vi "ImagerForFlowbit.vi"() -> ()   [LabVIEW 2011]
uses:
  <vilib>/Platform/TimedLoop/XDataNode/timing_clust.ctl
  <vilib>/Platform/TimedLoop/XDataNode/nitl_modes.ctl
  <vilib>/Platform/TimedLoop/XDataNode/wakeup.ctl
  <vilib>/Instr/_visa.llb/VISA Configure Serial Port (Instr).vi
  <vilib>/Platform/TimedLoop/XDataNode/XDataNode.xnode
  <vilib>/Platform/TimedLoop/XDataNode/XDNodeRunTimeDep.lvlib
  <vilib>/vision/NI_Vision_Development_Module.lvlib
panel:
  in  "热图":bool
  out "FramesPerStim":i32
  out "停止 4":bool
  in  "停止 3":bool
  in  "recording_temp":bool
  in  "datatype":enum16{"U8", "I16", "U32", "SGL"}(ring)=enum."SGL"
  out "Y Resolution":i32
  out "X Resolution":i32
  in  "frame_count":i32
  out "队列中元素数量":i32(slide) scale=0.0..100.0
  out "当前blk句柄":refnum<file>
  out "Recording":bool
  in  "bin_num":i32=25
  out "错误输出":errorcluster
  in  "BlkFolderPath":path=path "D:/Expt/test"
  out "循环持续时间":i64
  out "Image":T1(plugin-control)
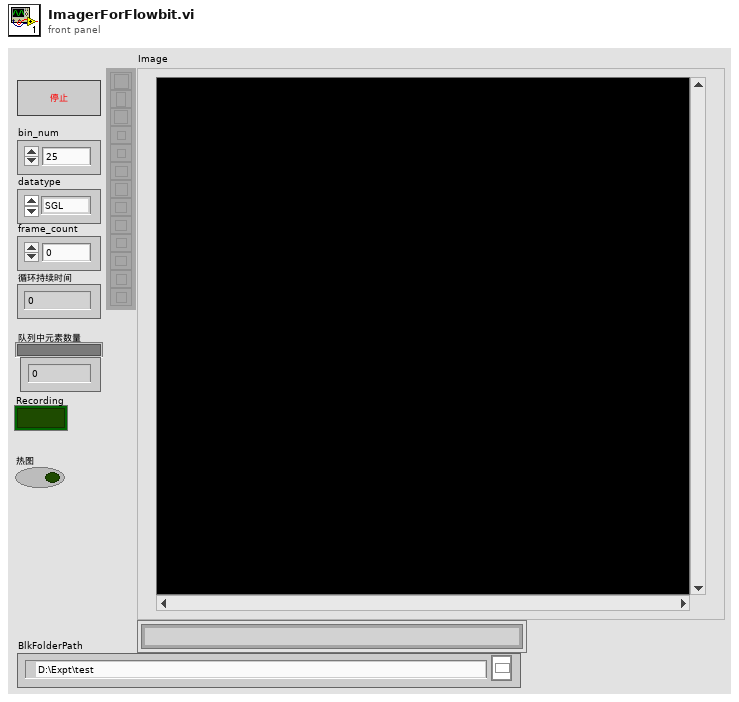
[diagram p1: front panel]
types:
  T1 = typedef "IMAQ Image.ctl" = refnum<image>
  T2 = typedef "Image Type" = u32
  T3 = enum16{"Disable External Trigger", "Enable External Trigger"}
  T4 = enum32{"Auto Detect", "RoadRunner", "Raven", "R64"}
  T5 = enum16{"open", "replace", "create", "open or create", "replace or create", "replace or create with confirmation"}
  T6 = typedef "XDNodeRunTimeDep.lvlib/timing_clust.ctl" = cluster{"Expected End [f-1]":u64, "Actual End [f-1]":u64, "Finished Late? [f-1]":bool, "Expected End [i-1]":u64, "Actual End [i-1]":u64, "Finished Late? [i-1]":bool, "Expected Start [i]":u64, "Actual Start [i]":u64, "Expected Start [f]":u64, "Actual Start [f]":u64, "Source Name":string, "Structure Name":string, "Period":i64, "Deadline":i64, "Offset":i64, "Start":i64, "Priority":i32, "Timeout":i32, "Mode":T7, "Wakeup Reason":T8, "Error":errorcluster, "Source Type":string, "Secondary Source Type":string, "Global End Time":u64, "Global Start Time":u64, "Frame Duration":u64, "Iteration Duration":u64, "Assigned CPU":i32, "I/O Scan Engine Mode":u32}
  T7 = typedef "XDNodeRunTimeDep.lvlib/nitl_modes.ctl" = enum32{"No Change", "Process missed periods, maintain original phase", "Discard missed periods, maintain original phase", "Process missed periods, ignore original phase", "Discard missed periods, ignore original phase"}
  T8 = typedef "XDNodeRunTimeDep.lvlib/wakeup.ctl" = enum32{"Normal", "Aborted", "Asynchronous wakeup", "Timing source error", "Timed loop error", "Timeout"}
  T9 = enum16{"big-endian, network order", "native, host order", "little-endian"}
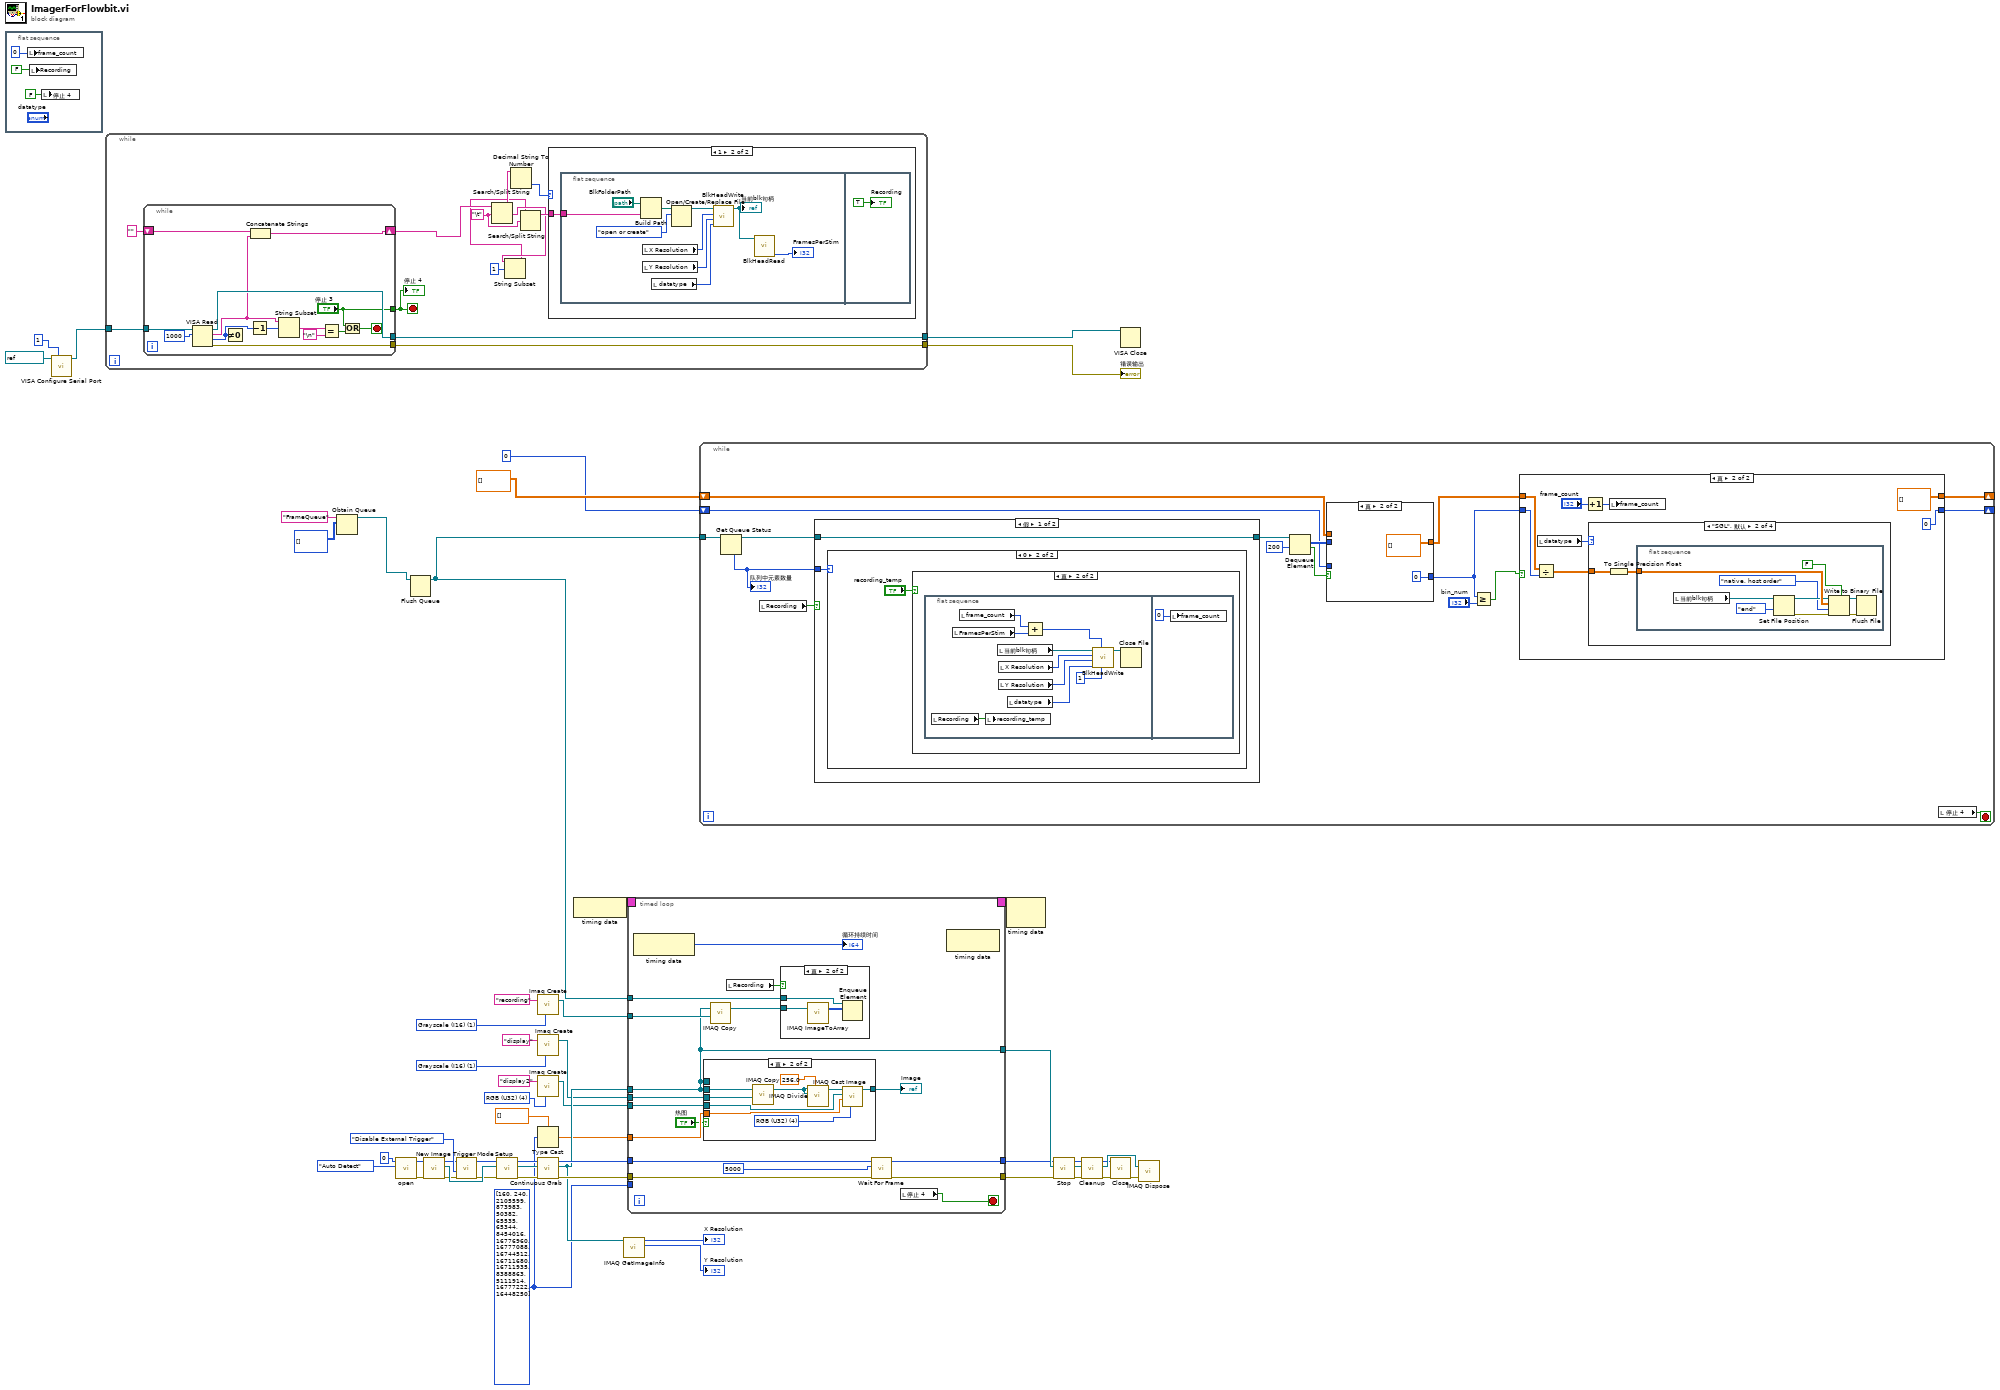
[diagram p0: block diagram]
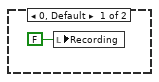
[diagram p2: hidden frame]
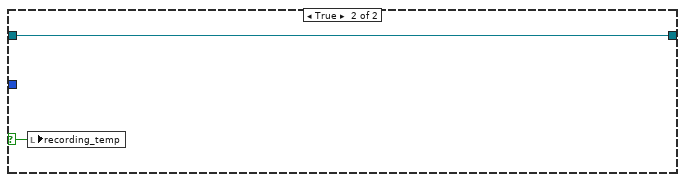
[diagram p7: hidden frame]
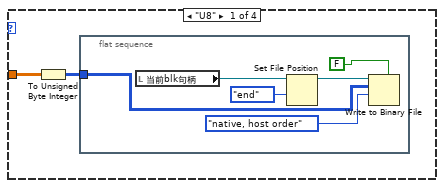
[diagram p9: hidden frame]
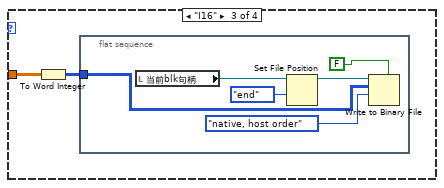
[diagram p10: hidden frame]
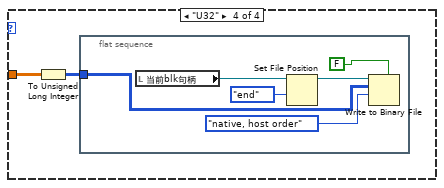
[diagram p11: hidden frame]
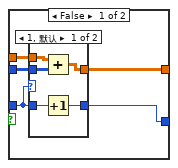
[diagram p12: hidden frame]
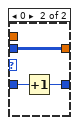
[diagram p13: hidden frame]
diagram:
  w5 = T2 4 items=["Grayscale (U8)", "Grayscale (I16)", "Grayscale (SGL)", "Complex (CSG)", "RGB (U32)", "HSL (U32)", "RGB (U64)", "Grayscale (U16)"] ("Image Type")
  w3 = u32[] [160, 240, 2105599, 873983, 50382, 65535, 65344, 8454016, 16776960, 16777088, 16744512, 16711680, 16711935, 8388863, 5111914, 16777222, 16448250] ("数组")
  w9 = T2 1 items=["Grayscale (U8)", "Grayscale (I16)", "Grayscale (SGL)", "Complex (CSG)", "RGB (U32)", "HSL (U32)", "RGB (U64)", "Grayscale (U16)"] ("Image Type")
  w24 = T2 1 items=["Grayscale (U8)", "Grayscale (I16)", "Grayscale (SGL)", "Complex (CSG)", "RGB (U32)", "HSL (U32)", "RGB (U64)", "Grayscale (U16)"] ("Image Type")
  n1 = flat-sequence {
    frame #0 {
      n2 = local write "frame_count"(0 ("frame_count")) -> ()
      n3 = local write "Recording"(FALSE ("Recording")) -> ()
      n4 = local write "停止 4"(FALSE ("停止 3")) -> ()
    }
  }
  n5 = call-poly "VISA Configure Serial Port"("VISA resource name"=refnum<visa-resource-name> "COM3", "timeout (10sec)"=u32 1) -> ("VISA resource name out"=w22:refnum<visa-resource-name>)  [unwired: 12 in, 1 out]
  n6 = while {
    tunnel: w22 -> [w68]
    tunnel: [w67] -> w20
    tunnel: [w66] -> w19
    stop <- w65 stop-if-true
    w62 = "\t"
    n7 = while {
      tunnel: w68 -> [w95]
      tunnel: [w94] -> w67
      tunnel: [w93] -> w66
      shift-right: [w86] -> w60
      shift-left: "" ("read buffer") -> [w92]
      tunnel: ["停止 3"] -> w65
      stop <- w84 stop-if-true
      n8 = VISA Read(VISA resource name=w95, byte count=u32 1000 ("字节总数")) -> (VISA resource name out=w93:refnum<visa-resource-name>, read buffer=w91:string, return count=w90:u32, error out=w94:errorcluster)  [unwired: 1 in]
      n9 = Not Equal To 0?(x=w90) -> ()  [unwired: 1 out]
      n10 = Decrement(x=w90) -> (x-1=w89:u32)
      n11 = Concatenate Strings(w92, w91) -> (w86:string)
      n12 = String Subset(string=w91, offset (0)=w89) -> (substring=w88:string)  [unwired: 1 in]
      n13 = Equal?(x=w88, y="\n") -> (x = y?=w85:bool)
      n14 = Or(x="停止 3", y=w85) -> (x .or. y?=w84:bool)
    }
    "停止 4" <- w65
    n15 = Search/Split String(string=w60, search string/char (-)=w62) -> (substring before match=w63:string, match + rest of string=w59:string)  [unwired: 1 in, 1 out]
    n16 = String Subset(string=w59, offset (0)=1 ("偏移量(0)")) -> (substring=w57:string)  [unwired: 1 in]
    n17 = Decimal String To Number(string=w63) -> (number=w64:i32)  [unwired: 2 in, 1 out]
    n18 = Search/Split String(string=w57, search string/char (-)=w62) -> (substring before match=w61:string)  [unwired: 1 in, 2 out]
    n19 = case shown="1" w64 {
      tunnel: w61 -> [_ w71]
      frame 0, Default {
        n20 = local write "Recording"(FALSE ("Recording")) -> ()
      }
      frame 1 {
        n21 = flat-sequence {
          tunnel: w71 -> [w75]
          frame #0 {
            n22 = Build Path(base path="BlkFolderPath", name or relative path=w75) -> (appended path=w79:path)
            n23 = local read "X Resolution"() -> (w78:i32)
            n24 = local read "Y Resolution"() -> (w77:i32)
            n25 = local read "datatype"() -> (w76:enum16{"U8", "I16", "U32", "SGL"})
            n26 = Open/Create/Replace File(file path (use dialog)=w79, operation (0:open)=T5."open or create" ("操作(0:open)")) -> (refnum out=w72:refnum<file>)  [unwired: 4 in, 2 out]
            n27 = call "BlkHeadWrite.vi"("datatype"=w76, "FrameHeight"=w77, "FrameWidth"=w78, "BlkFile"=w72) -> ("引用句柄输出"=w74:refnum<file>)  [unwired: 7 in]
            "当前blk句柄" <- w74
            n28 = call "BlkHeadRead.vi"("引用句柄"=w74) -> ("FramesPerStim"=→"FramesPerStim":i32)  [unwired: 5 in, 5 out]
          }
          frame #1 {
            "Recording" <- TRUE ("Recording")
          }
        }
      }
    }
  }
  "错误输出" <- w20
  n29 = Obtain Queue(name (unnamed)="FrameQueue" ("名称（未命名）"), element data type=i16[][] []) -> (queue out=w11:refnum<queue>)  [unwired: 3 in, 2 out]
  n30 = call <vilib>:"open.vi"("Board Type"=T4."Auto Detect", "Board Number"=u32 0) -> ("error out"=w42:errorcluster, "RefBrdOut"=w37:u32)  [unwired: 2 in, 5 out]
  n31 = Flush Queue(queue=w11) -> (queue out=w10:refnum<queue>)  [unwired: 1 in, 2 out]
  n32 = call <vilib>:"New Image.vi"("RefBrdIn"=w37, "error in"=w42) -> ("RefBrdOut"=w36:u32, "Image"=w51:T1, "error out"=w43:errorcluster)  [unwired: 6 in]
  n33 = call <vilib>:"Trigger Mode.vi"("RefBrdIn"=w36, "Trigger Mode"=T3."Disable External Trigger", "error in (no error)"=w43) -> ("RefBrdOut"=w35:u32, "error out"=w44:errorcluster)  [unwired: 6 in]
  n34 = call <vilib>:"Setup.vi"("error in"=w44, "Image In"=w51, "RefBrdIn"=w35) -> ("error out"=w39:errorcluster, "Image"=w40:T1, "RefBrdOut"=w34:u32)  [unwired: 6 in]
  n35 = call "Imaq Create"("Image Name"="recording", "Image Type"=w24) -> ("New Image"=w26:T1)  [unwired: 3 in, 1 out]
  n36 = call "Imaq Create"("Image Name"="display", "Image Type"=w9) -> ("New Image"=w7:T1)  [unwired: 3 in, 1 out]
  n37 = call "Imaq Create"("Image Name"="display2", "Image Type"=w5) -> ("New Image"=w4:T1)  [unwired: 3 in, 1 out]
  n38 = Type Cast(type=sgl[] [] ("单精度浮点"), x=w3) -> (*(type *) &x=w1:sgl[])
  n39 = call <vilib>:"Continuous Grab.vi"("error in (no error)"=w39, "Image In"=w40, "RefBrdIn"=w34) -> ("error out"=w38:errorcluster, "Image"=w14:T1, "RefBrdOut"=w33:u32)  [unwired: 6 in]
  n40 = node-c288() -> (w28:T6)
  n41 = call "IMAQ GetImageInfo"("Image"=w14) -> ("Y Resolution"=→"Y Resolution":i32, "X Resolution"=→"X Resolution":i32)  [unwired: 3 in, 6 out]
  n42 = timed-loop {
    tunnel: [w99] -> w50
    tunnel: [w113] -> w45
    tunnel: w14 -> [w99]
    tunnel: w38 -> [w112]
    tunnel: w33 -> [w111]
    tunnel: [w110] -> w32
    timing: w28 -> [_]
    timing-out: [_] -> w27
    tunnel: w26 -> [w104]
    tunnel: w10 -> [w108]
    tunnel: w7 -> [w102]
    tunnel: w3 -> [_]
    tunnel: w4 -> [w101]
    tunnel: w1 -> [w100]
    stop <- w105 stop-if-true
    n43 = node-c288() -> (→"循环持续时间":i64)  [unwired: 1 in]
    n44 = case shown="真" "热图" {
      tunnel: w102 -> [_ w122]
      tunnel: w99 -> [_ w120]
      tunnel: [w114 w119] -> w98
      tunnel: w101 -> [_ w117]
      tunnel: w100 -> [_ w116]
      tunnel: w99 -> [w114 _]
      frame False {
      }
      frame True {
        w118 = T2 4 items=["Grayscale (U8)", "Grayscale (I16)", "Grayscale (SGL)", "Complex (CSG)", "RGB (U32)", "HSL (U32)", "RGB (U64)", "Grayscale (U16)"] ("Image Type")
        n45 = call "IMAQ Copy"("Image Dst"=w122, "Image Src"=w120) -> ("Image Dst Out"=w121:T1)  [unwired: 4 in, 1 out]
        n46 = call "IMAQ Divide"("Image Src A"=w121, "Constant"=sgl 256.0, "Image Dst"=w121) -> ("Image Dst Out"=w115:T1)  [unwired: 4 in, 1 out]
        n47 = call "IMAQ Cast Image"("Image Type"=w118, "Lookup Table"=w116, "Image Dst"=w117, "Image Src"=w115) -> ("Image Dst Out"=w119:T1)  [unwired: 6 in, 1 out]
      }
    }
    "Image" <- w98
    n48 = call "IMAQ Copy"("Image Dst"=w104, "Image Src"=w99) -> ("Image Dst Out"=w103:T1)  [unwired: 4 in, 1 out]
    n49 = local read "Recording"() -> (w106:bool)
    n50 = case shown="真" w106 {
      tunnel: w108 -> [_ w126]
      tunnel: w103 -> [_ w124]
      frame False {
      }
      frame True {
        n51 = call "IMAQ ImageToArray"("Image"=w124) -> ("Image Pixels (I16)"=w125:i16[][])  [unwired: 3 in, 4 out]
        n52 = Enqueue Element(queue=w126, element=w125) -> ()  [unwired: 2 in, 3 out]
      }
    }
    n53 = call <vilib>:"Wait For Frame.vi"("error in (no error)"=w112, "Timeout (mS)"=u32 5000, "RefBrdIn"=w111) -> ("error out"=w113:errorcluster, "RefBrdOut"=w110:u32)  [unwired: 7 in]
    n54 = local read "停止 4"() -> (w105:bool)
    n55 = node-c288() -> ()  [unwired: 1 in, 1 out]
  }
  n56 = while {
    tunnel: w10 -> [w146]
    shift-right: [w139] -> _
    shift-left: sgl[][] [] -> [w143]
    shift-right: [w138] -> _
    shift-left: 0 ("加法记数") -> [w142]
    stop <- w133 stop-if-true
    n57 = Get Queue Status(queue=w146) -> (queue out=w136:refnum<queue>, # elements in queue=w131:i32)  [unwired: 2 in, 6 out]
    "队列中元素数量" <- w131
    n58 = local read "Recording"() -> (w135:bool)
    n59 = case shown="假" w135 {
      selector: w135 -> [_ w161]
      tunnel: w136 -> [w147 w162]
      tunnel: [w147 w162] -> w134
      tunnel: w131 -> [w148 _]
      frame False {
        n60 = case shown="0" w148 {
          frame 1, Default {
          }
          frame 0 {
            n61 = case shown="真" "recording_temp" {
              frame False {
              }
              frame True {
                n62 = flat-sequence {
                  frame #0 {
                    n63 = local read "Recording"() -> (w153:bool)
                    n64 = local read "FramesPerStim"() -> (w151:i32)
                    n65 = local read "frame_count"() -> (w152:i32)
                    n66 = local write "recording_temp"(w153) -> ()
                    n67 = local read "当前blk句柄"() -> (w156:refnum<file>)
                    n68 = local read "X Resolution"() -> (w159:i32)
                    n69 = local read "Y Resolution"() -> (w158:i32)
                    n70 = local read "datatype"() -> (w154:enum16{"U8", "I16", "U32", "SGL"})
                    n71 = Add(x=w152, y=w151) -> (x+y=w150:i32)
                    n72 = call "BlkHeadWrite.vi"("Stimuli"=1, "FramesPerStim"=w150, "datatype"=w154, "FrameHeight"=w158, "FrameWidth"=w159, "BlkFile"=w156) -> ("引用句柄输出"=w155:refnum<file>)  [unwired: 5 in]
                    n73 = Close File(refnum=w155) -> ()  [unwired: 1 in, 2 out]
                  }
                  frame #1 {
                    n74 = local write "frame_count"(0 ("frame_count")) -> ()
                  }
                }
              }
            }
          }
        }
      }
      frame True {
        n75 = local write "recording_temp"(w161) -> ()
      }
    }
    n76 = Dequeue Element(queue=w134, timeout in ms (-1)=200 ("超时毫秒(-1)")) -> (element=w144:i16[][], timed out?=w145:bool)  [unwired: 1 in, 2 out]
    n77 = case shown="真" w145 {
      tunnel: w144 -> [w212 _]
      tunnel: [w211 sgl[][] []] -> w141
      tunnel: w143 -> [w210 _]
      tunnel: w142 -> [w209 _]
      tunnel: [w208 0] -> w132
      frame False {
        n78 = case shown="1, 默认" w209 {
          tunnel: w212 -> [w217 w220]
          tunnel: [w215 w220] -> w211
          tunnel: w210 -> [w216 _]
          tunnel: w209 -> [w214 w219]
          tunnel: [w213 w218] -> w208
          frame 1, Default {
            n79 = Add(x=w216, y=w217) -> (x+y=w215:sgl[][])
            n80 = Increment(x=w214) -> (x+1=w213:i32)
          }
          frame 0 {
            n81 = Increment(x=w219) -> (x+1=w218:i32)
          }
        }
      }
      frame True {
      }
    }
    n82 = Greater Or Equal?(x=w132, y="bin_num") -> (x >= y?=w130:bool)
    n83 = case shown="真" w130 {
      tunnel: w141 -> [w164 w171]
      tunnel: [w164 sgl[][] []] -> w139
      tunnel: w132 -> [w163 w169]
      tunnel: [w163 0 ("加法记数")] -> w138
      frame False {
      }
      frame True {
        n84 = Divide(x=w171, y=w169) -> (x/y=w172:sgl[][])
        n85 = local read "datatype"() -> (w165:enum16{"U8", "I16", "U32", "SGL"})
        n86 = Increment(x="frame_count") -> (x+1=w166:i32)
        n87 = case shown="\"SGL\", 默认" w165 {
          tunnel: w172 -> [w174 w182 w193 w201]
          frame "U8" {
            n88 = To Unsigned Byte Integer(number=w174) -> (unsigned 8bit integer=w173:u8[][])
            n89 = flat-sequence {
              tunnel: w173 -> [w179]
              frame #0 {
                n90 = local read "当前blk句柄"() -> (w180:refnum<file>)
                n91 = Set File Position(refnum=w180, from (0:start)=enum16{"start", "end", "current"}."end" ("自（0:起始）")) -> (refnum out=w178:refnum<file>)  [unwired: 2 in, 1 out]
                n92 = Write to Binary File(file (use dialog)=w178, data=w179, 5:FALSE ("预置数组或字符串大小？(T)"), 9:T9."native, host order" ("字节顺序(0:big-endian, network order)")) -> ()  [unwired: 2 in, 3 out]
              }
            }
          }
          frame "SGL", Default {
            n93 = To Single Precision Float(number=w182) -> (single precision float=w181:sgl[][])
            n94 = flat-sequence {
              tunnel: w181 -> [w190]
              frame #0 {
                n95 = local read "当前blk句柄"() -> (w191:refnum<file>)
                n96 = Set File Position(refnum=w191, from (0:start)=enum16{"start", "end", "current"}."end" ("自（0:起始）")) -> (refnum out=w189:refnum<file>, error out=w183:errorcluster)  [unwired: 2 in]
                n97 = Write to Binary File(file (use dialog)=w189, data=w190, error in=w183, 5:FALSE ("预置数组或字符串大小？(T)"), 9:T9."native, host order" ("字节顺序(0:big-endian, network order)")) -> (refnum out=w185:refnum<file>, error out=w184:errorcluster)  [unwired: 1 in, 1 out]
                n98 = Flush File(refnum=w185, error in=w184) -> ()  [unwired: 2 out]
              }
            }
          }
          frame "I16" {
            n99 = To Word Integer(number=w193) -> (16bit integer=w192:i16[][])
            n100 = flat-sequence {
              tunnel: w192 -> [w198]
              frame #0 {
                n101 = local read "当前blk句柄"() -> (w199:refnum<file>)
                n102 = Set File Position(refnum=w199, from (0:start)=enum16{"start", "end", "current"}."end" ("自（0:起始）")) -> (refnum out=w197:refnum<file>)  [unwired: 2 in, 1 out]
                n103 = Write to Binary File(file (use dialog)=w197, data=w198, 5:FALSE ("预置数组或字符串大小？(T)"), 9:T9."native, host order" ("字节顺序(0:big-endian, network order)")) -> ()  [unwired: 2 in, 3 out]
              }
            }
          }
          frame "U32" {
            n104 = To Unsigned Long Integer(number=w201) -> (unsigned 32bit integer=w200:u32[][])
            n105 = flat-sequence {
              tunnel: w200 -> [w206]
              frame #0 {
                n106 = local read "当前blk句柄"() -> (w207:refnum<file>)
                n107 = Set File Position(refnum=w207, from (0:start)=enum16{"start", "end", "current"}."end" ("自（0:起始）")) -> (refnum out=w205:refnum<file>)  [unwired: 2 in, 1 out]
                n108 = Write to Binary File(file (use dialog)=w205, data=w206, 5:FALSE ("预置数组或字符串大小？(T)"), 9:T9."native, host order" ("字节顺序(0:big-endian, network order)")) -> ()  [unwired: 2 in, 3 out]
              }
            }
          }
        }
        n109 = local write "frame_count"(w166) -> ()
      }
    }
    n110 = local read "停止 4"() -> (w133:bool)
  }
  n111 = node-c288(w27) -> ()  [unwired: 1 out]
  n112 = call <vilib>:"Stop.vi"("error in (no error)"=w45, "Image In"=w50, "RefBrdIn"=w32) -> ("error out"=w46:errorcluster, "Image"=w49:T1, "RefBrdOut"=w31:u32)  [unwired: 6 in]
  n113 = call <vilib>:"Cleanup.vi"("error in (no error)"=w46, "Image In"=w49, "RefBrdIn"=w31) -> ("error out"=w47:errorcluster, "Image"=w48:T1, "RefBrdOut"=w30:u32)  [unwired: 6 in]
  n114 = call <vilib>:"Close.vi"("error in (no error)"=w47, "RefBrdIn"=w30) -> ("error out"=w29:errorcluster)  [unwired: 8 in, 1 out]
  n115 = VISA Close(VISA resource name=w19) -> ()  [unwired: 1 in, 1 out]
  n116 = call "IMAQ Dispose"("Image"=w48, "error in (no error)"=w29) -> ()  [unwired: 4 in, 1 out]
